vi "FunctionalGlobal.vi"(6 "Set?":bool, 8 "ErrorIn":errorcluster, 11 "ClusterIn":T1={"MainQ"=refnum, "User"={"Lvl"=enum."Admin", "Pwd"=""}, "Stat"={"SysState"=enum."Init", "TrackRate"=FALSE, "AutoCentr"=FALSE}, "Paths"={"CfgFile"=path "", "LogFolder"=path "", "LogFile"=path "", "NAS path"=path "", "ThreshFile"=path "", "RedunFolder"=path ""}, "HW"={"All_FPGAs"={"1"={"Ref"=refnum, "Cal"={"Fine"=0.0, "Coarse_"=-24999000.0}, "Beac"={"Fine"=-462.63345195729516, "Coarse_"=-24999000.0}, "EnableStep1"=FALSE, "Enable"={"FreqShiftEnable"=TRUE, "Step4Enable"=TRUE, "Step5Enable"=TRUE, "Step6Enable"=TRUE, "Step7Enable"=TRUE}, "FlushQ"=TRUE, "Offset"=0.000213623046875, "Scale_NoiseFloor"=4194303.0, "Scale_In_RT"=1.0, "ScaleMeasurement"=10000.0, "Scale_Step1"=4194303.0, "Scale"={"Scale_Step4"=10.0, "Scale_Step5"=1.0, "Scale_Step6"=1.0, "Scale_Step7"=1.0}}, "2"={"Target"=enum."1", "Channel"=enum."4", "Ref1"=refnum, "Ref2"=refnum}, "3"={"Target"=enum."1", "Channel"=enum."4", "Ref1"=refnum, "Ref2"=refnum}, "4"={"Target"=enum."1", "Channel"=enum."4", "Ref1"=refnum, "Ref2"=refnum}}}}) -> (0 "ErrorOut":errorcluster, 3 "ClusterOut":T1={"MainQ"=refnum, "User"={"Lvl"=enum."Admin", "Pwd"=""}, "Stat"={"SysState"=enum."Init", "TrackRate"=FALSE, "AutoCentr"=FALSE}, "Paths"={"CfgFile"=path "", "LogFolder"=path "", "LogFile"=path "", "NAS path"=path "", "ThreshFile"=path "", "RedunFolder"=path ""}, "HW"={"All_FPGAs"={"1"={"Ref"=refnum, "Cal"={"Fine"=0.0, "Coarse_"=-24999000.0}, "Beac"={"Fine"=-462.63345195729516, "Coarse_"=-24999000.0}, "EnableStep1"=FALSE, "Enable"={"FreqShiftEnable"=TRUE, "Step4Enable"=TRUE, "Step5Enable"=TRUE, "Step6Enable"=TRUE, "Step7Enable"=TRUE}, "FlushQ"=TRUE, "Offset"=0.000213623046875, "Scale_NoiseFloor"=4194303.0, "Scale_In_RT"=1.0, "ScaleMeasurement"=10000.0, "Scale_Step1"=4194303.0, "Scale"={"Scale_Step4"=10.0, "Scale_Step5"=1.0, "Scale_Step6"=1.0, "Scale_Step7"=1.0}}, "2"={"Target"=enum."1", "Channel"=enum."4", "Ref1"=refnum, "Ref2"=refnum}, "3"={"Target"=enum."1", "Channel"=enum."4", "Ref1"=refnum, "Ref2"=refnum}, "4"={"Target"=enum."1", "Channel"=enum."4", "Ref1"=refnum, "Ref2"=refnum}}}})   [LabVIEW 2018]
doc: "Use an uninitialized shift register to store <B>ClusterIn</B> as a functional global variable. Note that this VI can be modified to handle any data type and is an effective way to pass data between different parts of the application. A functional global acts largtely like a global variable, but has the distinct advantage of forcing data flow, allowing for internal calculations and with the appropriate entrant/re-entrant configuration, ensure that the possibility of race condition is reduced (not impossible!).\n\nIf <B>Set?</B> is True, <B>ClusterIn</B> replaces the previously stored value. \n\nIf <B>Set?</B> is False, the currently stored value remains unchanged and <B>ClusterIn</B> is ignored.\n\nCopyright © 2011 Epimedia, Inc. All Rights Reserved.\n\nThe Epimedia Application Library is Copyright © 2009-2011 Epimedia, Inc. \nAll Rights Reserved. Used under license."
uses:
  Controls/PathsCluster.ctl
  Controls/UserLevelEnum.ctl
  Controls/Clusts/AdminCluster.ctl
  Controls/MasterCluster.ctl
  Queue/MainQueueElements.ctl
  Controls/SystemStatusCluster.ctl
  Controls/HWCluster.ctl
  Controls/SystemStateEnum.ctl
  Controls/Clusts/FreqShift.ctl
  Controls/Clusts/FPGA_Config_Clust.ctl
  Controls/Clusts/All_FPGAs_Config.ctl
  Controls/Enums/TargetNumber.ctl
panel:
  # "Copyright © 2011 Epimedia, Inc. All Rights Reserved.\n\nThe Epimedia Application Library is Copyright © 2009-2011 Epimedia, Inc. \nAll Rights Reserved. Used under license."
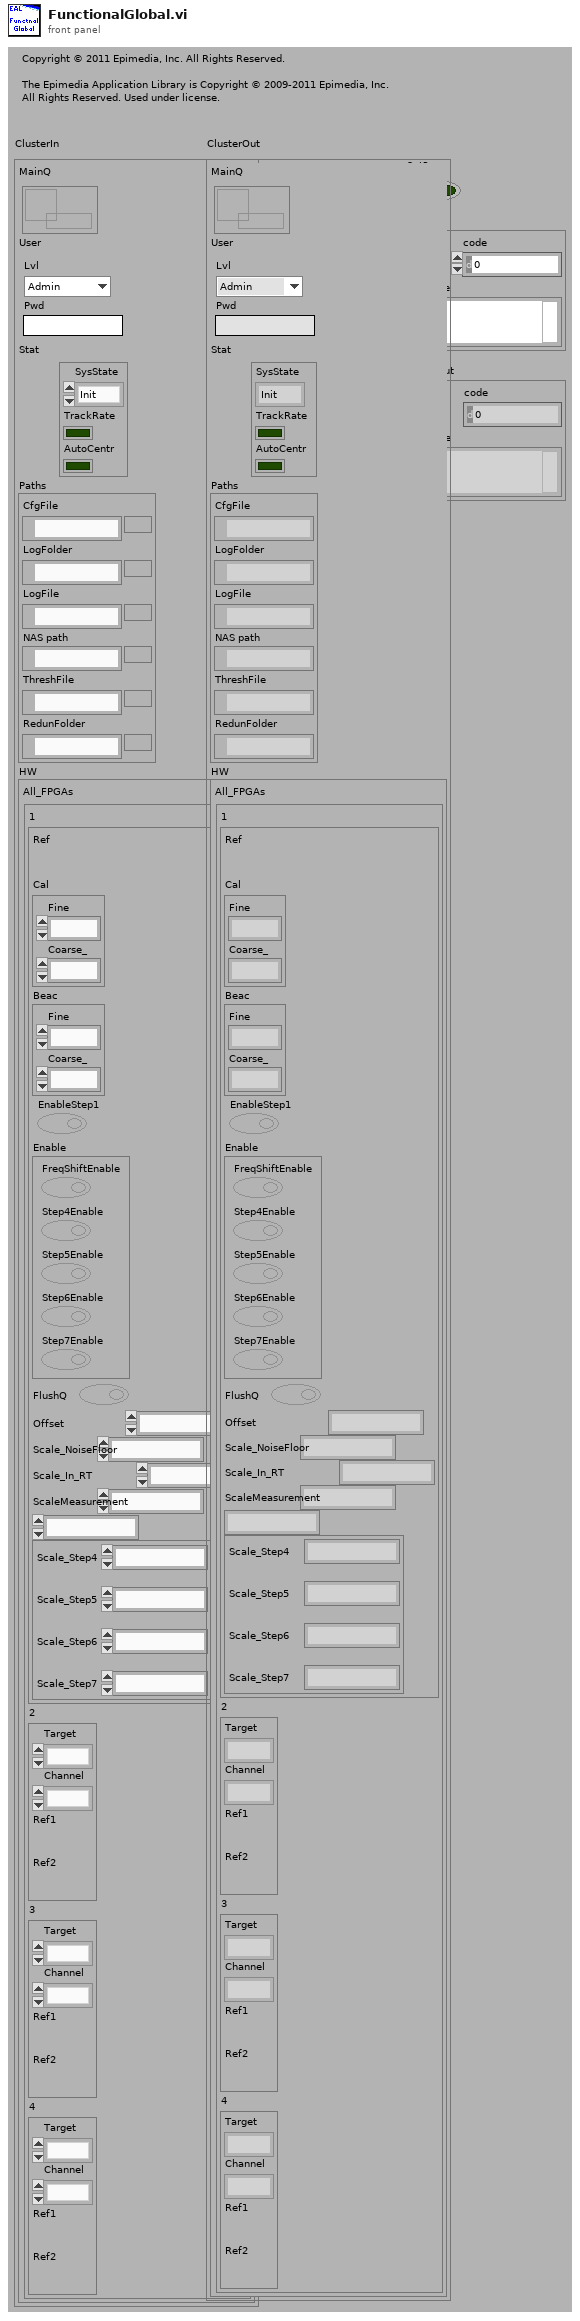
[diagram p1: front panel]
types:
  T1 = typedef "MasterCluster.ctl" = cluster{"MainQ":refnum<queue>, "User":T2, "Stat":T4, "Paths":T6, "HW":T7}
  T2 = typedef "AdminCluster.ctl" = cluster{"Lvl":T3, "Pwd":string}
  T3 = typedef "UserLevelEnum.ctl" = enum16{"Admin", "Operator"}
  T4 = typedef "SystemStatusCluster.ctl" = cluster{"SysState":T5, "TrackRate":bool, "AutoCentr":bool}
  T5 = typedef "SystemStateEnum.ctl" = enum16{"Init", "Idle", "Running", "System Fault", "System Error", "Exit"}
  T6 = typedef "PathsCluster.ctl" = cluster{"CfgFile":path, "LogFolder":path, "LogFile":path, "NAS path":path, "ThreshFile":path, "RedunFolder":path}
  T7 = typedef "HWCluster.ctl" = cluster{"All_FPGAs":T8}
  T8 = typedef "All_FPGAs_Config.ctl" = cluster{"1":T9, "2":T11, "3":T11, "4":T11}
  T9 = typedef "FPGA_Config_Clust.ctl" = cluster{"Ref":refnum<k20>, "Cal":T10, "Beac":T10, "EnableStep1":bool, "Enable":cluster{"FreqShiftEnable":bool, "Step4Enable":bool, "Step5Enable":bool, "Step6Enable":bool, "Step7Enable":bool}, "FlushQ":bool, "Offset":fxp<+/-,16,1>, "Scale_NoiseFloor":fxp<+/-,23,23>, "Scale_In_RT":ext, "ScaleMeasurement":fxp<+/-,23,23>, "Scale_Step1":fxp<+/-,23,23>, "Scale":cluster{"Scale_Step4":fxp<+/-,23,23>, "Scale_Step5":fxp<+/-,23,23>, "Scale_Step6":fxp<+/-,23,23>, "Scale_Step7":fxp<+/-,23,23>}}
  T10 = typedef "FreqShift.ctl" = cluster{"Fine":dbl, "Coarse_":dbl}
  T11 = typedef "FPGA_Config_Clust.ctl" = cluster{"Target":T12, "Channel":T12, "Ref1":refnum<k20>, "Ref2":refnum<k20>}
  T12 = typedef "TargetNumber.ctl" = enum16{"1", "2", "3", "4"}
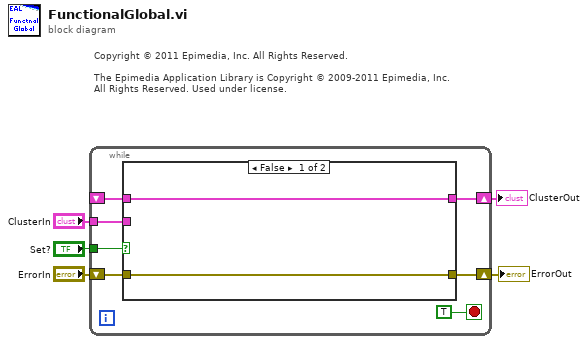
[diagram p0: block diagram]
diagram:
  # "Copyright © 2011 Epimedia, Inc. All Rights Reserved.\n\nThe Epimedia Application Library is Copyright © 2009-2011 Epimedia, Inc. \nAll Rights Reserved. Used under license."
  n1 = while {
    shift-right: [w11] -> w5
    shift-left: "ErrorIn" -> [w10]
    shift-right: [w8] -> w3
    shift-left: _ -> [w6]
    tunnel: "ClusterIn" -> [w9]
    tunnel: "Set?" -> [w7]
    stop <- TRUE stop-if-true
    n2 = case shown="False" w7 {
      tunnel: [w13 w16] -> w11
      tunnel: w10 -> [w13 w16]
      tunnel: w9 -> [_ w15]
      tunnel: [w14 w15] -> w8
      tunnel: w6 -> [w14 _]
      frame False {
      }
      frame True {
      }
    }
  }
  "ErrorOut" <- w5
  "ClusterOut" <- w3
